vi "RichToFlatnixnet_grpc_ReadSignalWaveformRequest.vi"(5 "OutputClusterType":T1, 11 "InputCluster":T4) -> (3 "OutputCluster":T1)   [LabVIEW 2025, in "grpc-xnet_client.lvlib"]
uses:
  grpc-xnet_client.lvlib
  nixnet_grpc_ReadSignalWaveformRequest.ctl
  nixnet_grpc_ReadSignalWaveformRequest_timeout_enum/nixnet_grpc_ReadSignalWaveformRequest_timeout_enum.lvclass
  nidevice_grpc_Session.ctl
  nixnet_grpc_ReadSignalWaveformRequest_Flat.ctl
  nidevice_grpc_Session_Flat.ctl
  nixnet_grpc_TimeOut.ctl
  nixnet_grpc_ReadSignalWaveformRequest_timeout_enum/nixnet_grpc_ReadSignalWaveformRequest_timeout_enum.lvclass/nixnet_grpc_ReadSignalWaveformRequest_timeout_enum.ctl
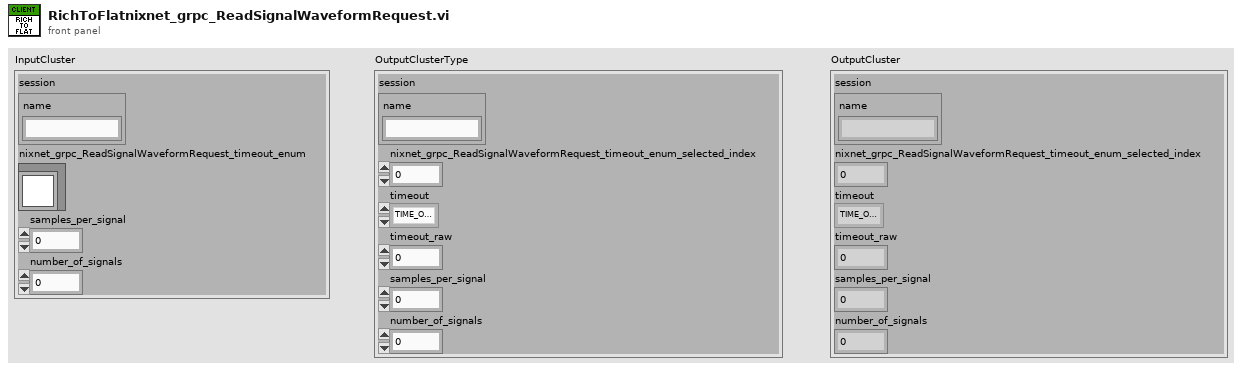
[diagram p1: front panel]
types:
  T1 = typedef "grpc-xnet_client.lvlib/nixnet_grpc_ReadSignalWaveformRequest_Flat.ctl" = cluster{"session":T2, "nixnet_grpc_ReadSignalWaveformRequest_timeout_enum_selected_index":i32, "timeout":T3, "timeout_raw":dbl, "samples_per_signal":u32, "number_of_signals":u32}
  T2 = typedef "grpc-xnet_client.lvlib/nidevice_grpc_Session_Flat.ctl" = cluster{"name":string}
  T3 = typedef "grpc-xnet_client.lvlib/nixnet_grpc_TimeOut.ctl" = enum32{"TIME_OUT_NONE", "TIME_OUT_INFINITE"}
  T4 = typedef "grpc-xnet_client.lvlib/nixnet_grpc_ReadSignalWaveformRequest.ctl" = cluster{"session":T5, "nixnet_grpc_ReadSignalWaveformRequest_timeout_enum":refnum<class "nixnet_grpc_ReadSignalWaveformRequest_timeout_enum.lvclass">, "samples_per_signal":u32, "number_of_signals":u32}
  T5 = typedef "grpc-xnet_client.lvlib/nidevice_grpc_Session.ctl" = cluster{"name":string}
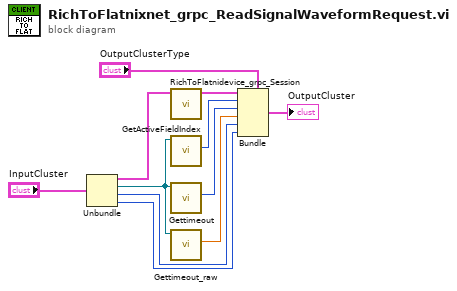
[diagram p0: block diagram]
diagram:
  n1 = Unbundle "Unbundle"("InputCluster") -> ("session"=w8:T5, "nixnet_grpc_ReadSignalWaveformRequest_timeout_enum"=w6:refnum<class "nixnet_grpc_ReadSignalWaveformRequest_timeout_enum.lvclass">, "samples_per_signal"=w2:u32, "number_of_signals"=w1:u32)
  n2 = call "RichToFlatnidevice_grpc_Session.vi"("InputCluster"=w8) -> ("OutputCluster"=w7:T2)  [unwired: 10 in]
  n3 = call "GetActiveFieldIndex.vi"("OneOfTemplate in"=w6) -> ("Active Field Index"=w5:i32)  [unwired: 8 in, 2 out]
  n4 = call "Gettimeout.vi"("OneOfTemplate in"=w6) -> ("Get_Val"=w4:T3)  [unwired: 8 in, 2 out]
  n5 = call "Gettimeout_raw.vi"("OneOfTemplate in"=w6) -> ("Get_Val"=w3:dbl)  [unwired: 8 in, 2 out]
  n6 = Bundle "Bundle"(cluster="OutputClusterType", "session"=w7, "nixnet_grpc_ReadSignalWaveformRequest_timeout_enum_selected_index"=w5, "timeout"=w4, "timeout_raw"=w3, "samples_per_signal"=w2, "number_of_signals"=w1) -> (→"OutputCluster":T1)
